vi "Test Config File.vi"(8 "error in (no error)":errorcluster, 10 "Test file?":bool, 11 "appended path in":path) -> (0 "error out":errorcluster, 3 "appended path out":path)   [LabVIEW 2018]
doc: "This VI tests the configuration file with the unit test included in the File Config class. \nIt uses a Dynamic reference to access it, so the class does not have to be loaded when this VI runs. Therefore, we don't need to have the robot code in the computer if we are just going to use the DS and Dashboard."
uses:
  <vilib>/Utility/sysdir.llb/System Directory Type.ctl
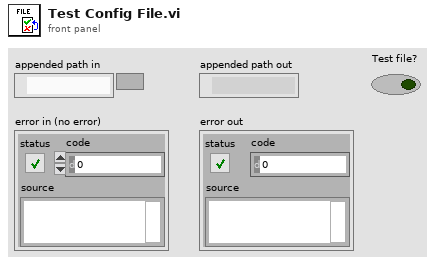
[diagram p1: front panel]
types:
  T1 = typedef "System Directory Type.ctl" = i32
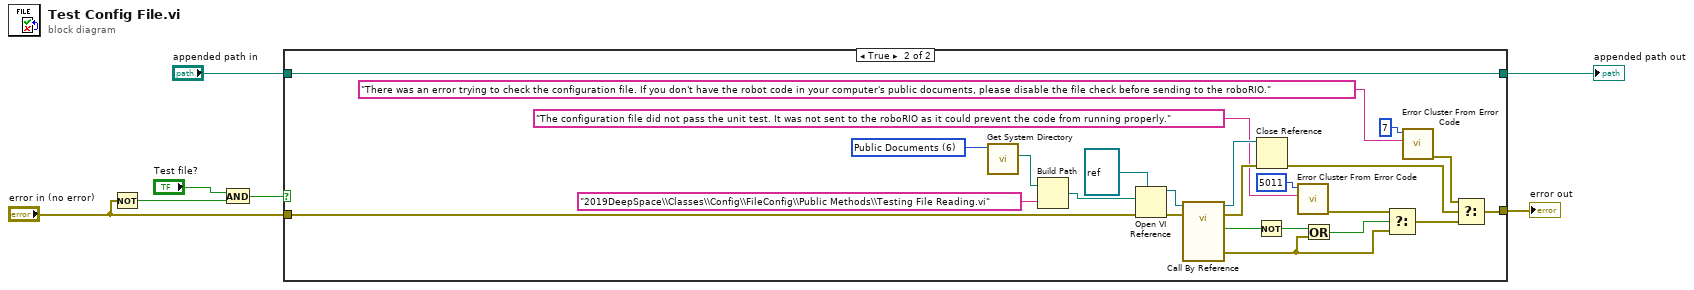
[diagram p0: block diagram]
diagram:
  n1 = Not(x="error in (no error)") -> (.not. x?=w3:bool)
  n2 = And(x="Test file?", y=w3) -> (x .and. y?=w4:bool)
  n3 = case shown="True" w4 {
    tunnel: [w9 w33] -> w5
    tunnel: "appended path in" -> [w9 w33]
    tunnel: [w8 w15] -> w7
    tunnel: "error in (no error)" -> [w8 w10]
    frame False {
    }
    frame True {
      w27 = T1 6 items=["User Home"=0, "User Desktop"=1, "User Documents"=2, "User Application Data"=3, "User Preferences"=4, "User Temporary"=5, "Public Documents"=6, "Public Application Data"=7, "Public Preferences"=8, "Public Cache"=13, "System Core Libraries"=9, "System Installed Libraries"=10, "Application Files"=11, "Boot Volume Root"=12] ("system directory type")
      n4 = call <vilib>:"Get System Directory.vi"("system directory type"=w27) -> ("system directory"=w25:path)  [unwired: 10 in]
      n5 = Build Path(base path=w25, name or relative path="2019DeepSpace\\Classes\\Config\\FileConfig\\Public Methods\\Testing File Reading.vi") -> (appended path=w26:path)
      n6 = Open VI Reference(type specifier VI Refnum (for type only)=refnum<vi> refnum, vi path=w26, error in (no error)=w10) -> (vi reference=w29:refnum<vi>, error out=w32:errorcluster)  [unwired: 3 in]
      n7 = call-by-ref "?"(reference=w29, error in=w32) -> (reference out=w31:refnum<vi>, error out=w30:errorcluster, 0:"error out"=w17:errorcluster, "Test result"=w22:bool)  [unwired: 10 in]
      n8 = Not(x=w22) -> (.not. x?=w20:bool)
      n9 = Close Reference(reference=w31, error in (no error)=w30) -> (error out=w14:errorcluster)
      n10 = call <vilib>:"Error Cluster From Error Code.vi"("error message (\"\")"="The configuration file did not pass the unit test. It was not sent to the roboRIO as it could prevent the code from running properly." ("error message (\"\")"), "error code (0)"=5011) -> ("error out"=w23:errorcluster)  [unwired: 7 in]
      n11 = Or(x=w20, y=w17) -> (x .or. y?=w21:bool)
      n12 = Select(t=w23, s=w21, f=w17) -> (s? t:f=w16:errorcluster)
      n13 = call <vilib>:"Error Cluster From Error Code.vi"("error message (\"\")"="There was an error trying to check the configuration file. If you don't have the robot code in your computer's public documents, please disable the file check before sending to the roboRIO." ("error message (\"\")"), "error code (0)"=7) -> ("error out"=w13:errorcluster)  [unwired: 7 in]
      n14 = Select(t=w13, s=w14, f=w16) -> (s? t:f=w15:errorcluster)
    }
  }
  "error out" <- w7
  "appended path out" <- w5
